vi "kalmanBall.vi"(1 "Detection Ball \nArray":T1[](array[typedef]), 2 "Life Time":dbl=2.0, 3 "Time Stamp 2":timestamp=timestamp(3583818425.330139 s since 1904-01-01), 5 "error in (no error)":errorcluster) -> (15 "balls":T1[](array[typedef]), 19 "error out":errorcluster)   [LabVIEW 2023, in "Vision.lvclass"]
uses:
  Vision.lvclass
  Old vision/Controls/SSL Detection Ball.ctl
  <vilib>/Analysis/Matrix/Datatypes/RealMatrix.ctl
  <vilib>/Analysis/Matrix/NI_Matrix.lvlib
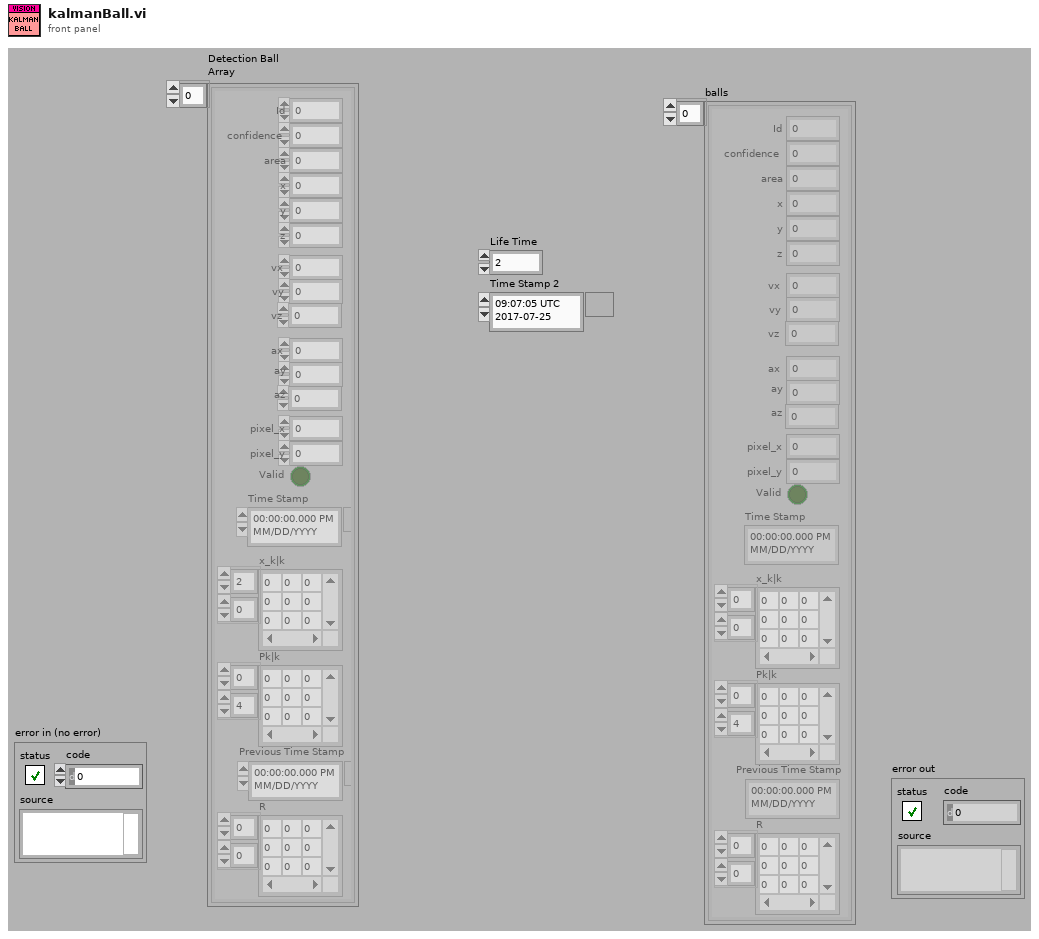
[diagram p1: front panel]
types:
  T1 = typedef "SSL Detection Ball.ctl" = cluster{"x":sgl, "area":u32, "confidence":sgl, "y":sgl, "z":sgl, "pixel_x":sgl, "pixel_y":sgl, "Valid":bool, "Time Stamp":timestamp, "x_k|k":T2, "Pk|k":T2, "Id":u32, "Previous Time Stamp":timestamp, "R":T2, " vx":sgl, "vy":dbl, "vz":dbl, " ax":sgl, "ay":dbl, "az":dbl}
  T2 = typedef "NI_Matrix.lvlib/RealMatrix.ctl" = dbl[][]
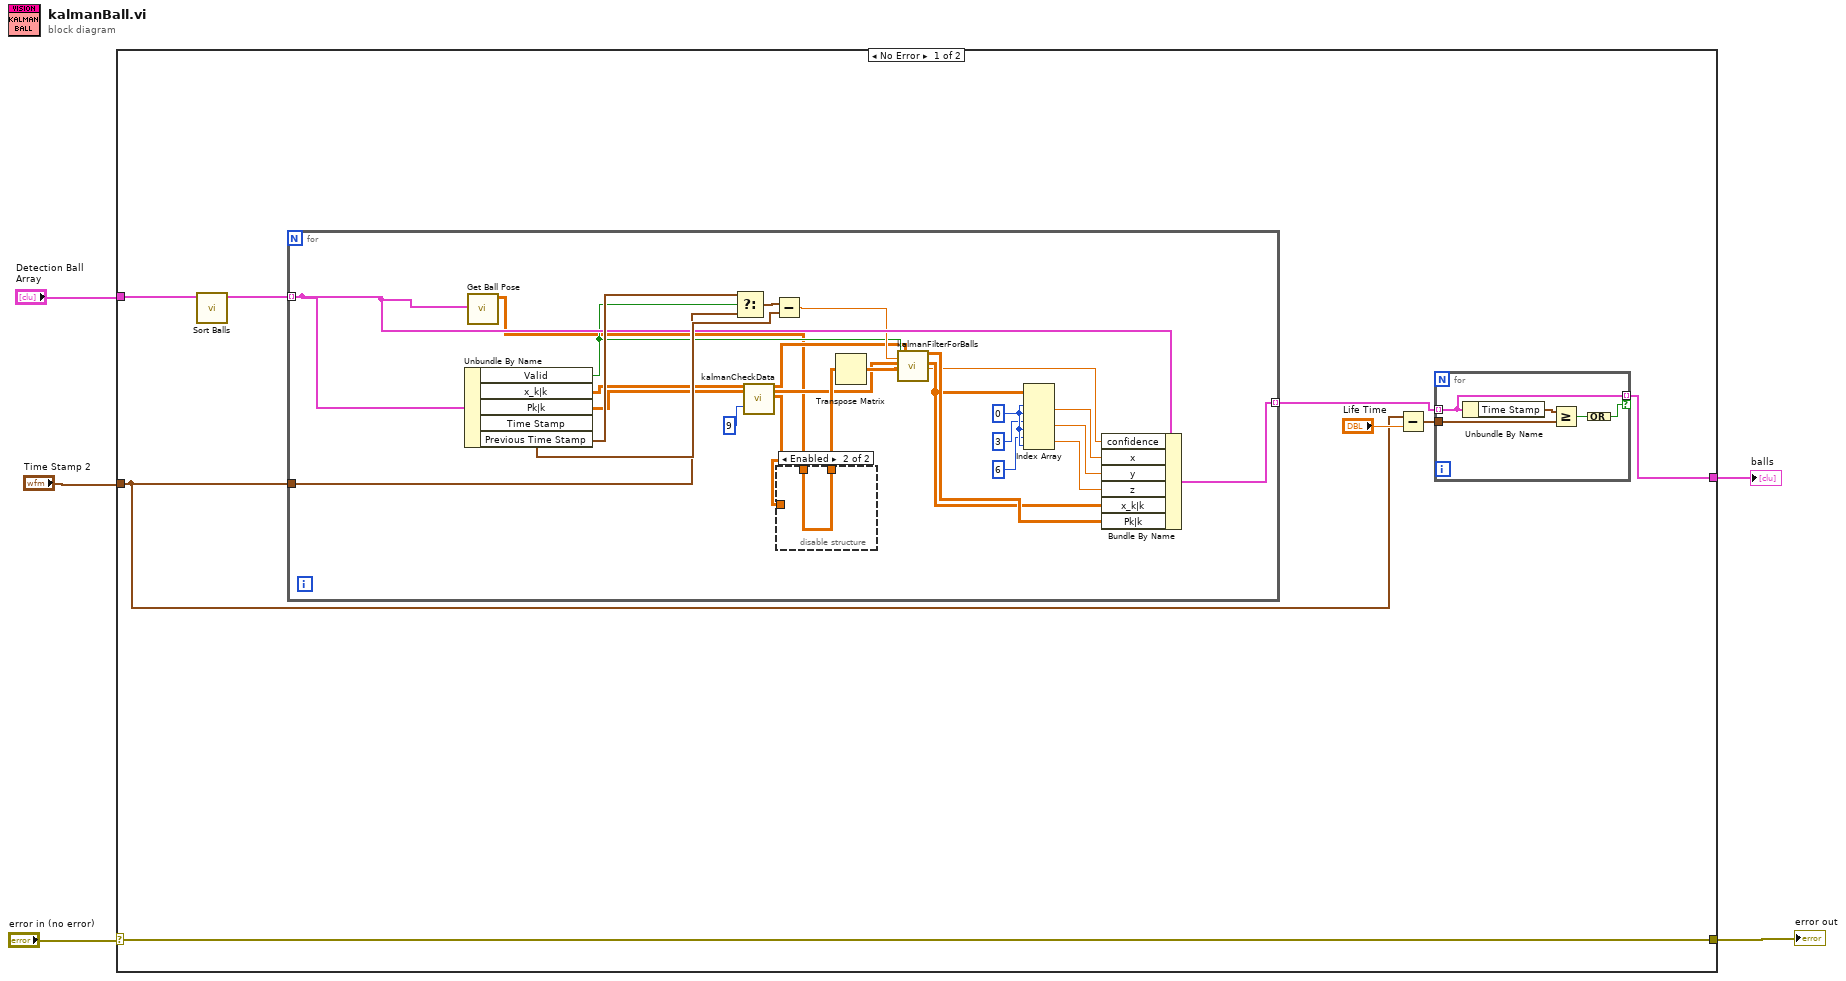
[diagram p0: block diagram]
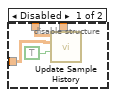
[diagram p2: hidden frame]
diagram:
  n1 = case shown="No Error" "error in (no error)" {
    selector: "error in (no error)" -> [w13 w50]
    tunnel: [w13 w50] -> w4
    tunnel: [w8 _] -> w3
    tunnel: "Time Stamp 2" -> [w7 _]
    tunnel: "Detection Ball \nArray" -> [w6 _]
    frame No Error {
      n2 = call "Sort Balls.vi"("Detection Ball \nArray"=w6) -> ("Sorted Detection Ball \nArray"=w9:T1[])  [unwired: 10 in]
      n3 = for {
        tunnel: w9 -> [w36] mode=indexing
        tunnel: [w37] -> w10 mode=indexing
        tunnel: w7 -> [w42]
        w40 = 0 ("index (row)")
        n4 = Unbundle By Name(w36) -> ("Valid"=w33:bool, "x_k|k"=w23:T2, "Pk|k"=w24:T2, "Time Stamp"=w43:timestamp, "Previous Time Stamp"=w44:timestamp)
        n5 = call "Get Ball Pose.vi"("Detection Ball"=w36) -> ("Pose"=w19:T2)  [unwired: 10 in]
        n6 = Select(t=w43, s=w33, f=w42) -> (s? t:f=w41:timestamp)
        n7 = call "kalmanCheckData.vi"("x_k"=w23, "Pk"=w24, "Variance Memory"=9) -> ("x_k out"=w22:T2, "Pk out"=w20:T2, "R out"=w21:T2)  [unwired: 13 in, 1 out]
        n8 = Subtract(x=w41, y=w44) -> (x-y=w35:dbl)
        n9 = disable-structure shown="Enabled" {
          disable-tunnel: [w47 w49] -> w30
          disable-tunnel: w19 -> [w46 w49]
          disable-tunnel: w21 -> [w45 _]
          frame Disabled {
            n10 = call "Update Sample History.vi"("Ball?"=TRUE, "R in"=w45, "Sample"=w46) -> ("Sample Unwrapped"=w47:T2)  [unwired: 6 in, 2 out]
          }
          frame Enabled {
          }
        }
        n11 = Transpose Matrix(1:w30) -> (0:w29:T2)
        n12 = call "kalmanFilterForBalls.vi"("Use Observation"=w33, "intervalo"=w35, "Pk-1|k-1"=w20, "z_k"=w29, "x_k-1|k-1"=w22) -> ("Pk|k out"=w34:T2, "x_k|k out"=w32:T2, "Conf"=w31:dbl)  [unwired: 11 in, 1 out]
        n13 = Index Array(array=w32, index (row) #1=w40, index (col) #1=w40, index (row) #2=3 ("disabled index (col)"), index (col) #2=w40, index (row) #3=6 ("disabled index (col)"), index (col) #3=w40) -> (element #1=w28:dbl, element #2=w27:dbl, element #3=w26:dbl)
        n14 = Bundle By Name(cluster=w36, "confidence"=w31, "x"=w28, "y"=w27, "z"=w26, "x_k|k"=w32, "Pk|k"=w34) -> (w37:T1)
      }
      n15 = Subtract(x=w7, y="Life Time") -> (x-y=w11:timestamp)
      n16 = for {
        tunnel: w10 -> [w18] mode=indexing
        tunnel: [w18] -> w8 mode=indexing if=w17
        tunnel: w11 -> [w15]
        n17 = Unbundle By Name(w18) -> ("Time Stamp"=w16:timestamp)
        n18 = Greater Or Equal?(x=w16, y=w15) -> (x >= y?=w14:bool)
        n19 = Compound Arithmetic op=OR(w14) -> (w17:bool)
      }
    }
    frame Error {
    }
  }
  "error out" <- w4
  "balls" <- w3
